vi "ti2_home_fgv.vi"(8 "Init?":bool, 9 "Y Init  (um)":dbl format="%#_13g", 10 "X Init (um)":dbl format="%#_13g") -> (1 "Y (um) 3":dbl, 2 "X (um) 2":dbl)   [LabVIEW 2018, in "ti2lv.lvlib"]
uses:
  ti2lv.lvlib
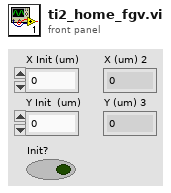
[diagram p1: front panel]
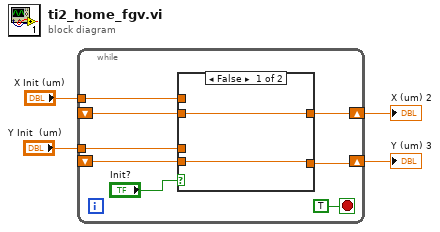
[diagram p0: block diagram]
diagram:
  n1 = while {
    shift-right: [w10] -> w4
    shift-left: _ -> [w11]
    shift-right: [w8] -> w3
    shift-left: _ -> [w9]
    tunnel: "Y Init  (um)" -> [w6]
    tunnel: "X Init (um)" -> [w5]
    stop <- TRUE stop-if-true
    n2 = case shown="False" "Init?" {
      tunnel: w11 -> [w14 _]
      tunnel: [w14 w15] -> w10
      tunnel: [w13 w16] -> w8
      tunnel: w9 -> [w13 _]
      tunnel: w6 -> [_ w16]
      tunnel: w5 -> [_ w15]
      frame False {
      }
      frame True {
      }
    }
  }
  "X (um) 2" <- w4
  "Y (um) 3" <- w3
